vi "S2C_Access_ManageUpdate.vi"(8 "Error In":errorcluster, 10 "Coords":cluster{"Row":i32, "Column":i32}, 11 "ItemTag":string) -> (0 "Error Out":errorcluster)   [LabVIEW 2015]
uses:
  S2C_Access_Globals.vi
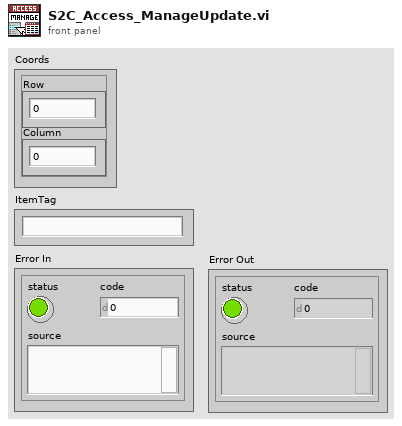
[diagram p1: front panel]
types:
  T1 = cluster{"ItemNames[0]":string, "ItemNames[1]":string, "ItemNames[2]":string}
  T2 = cluster{"[0]":string, "[1]":string, "[2]":string}
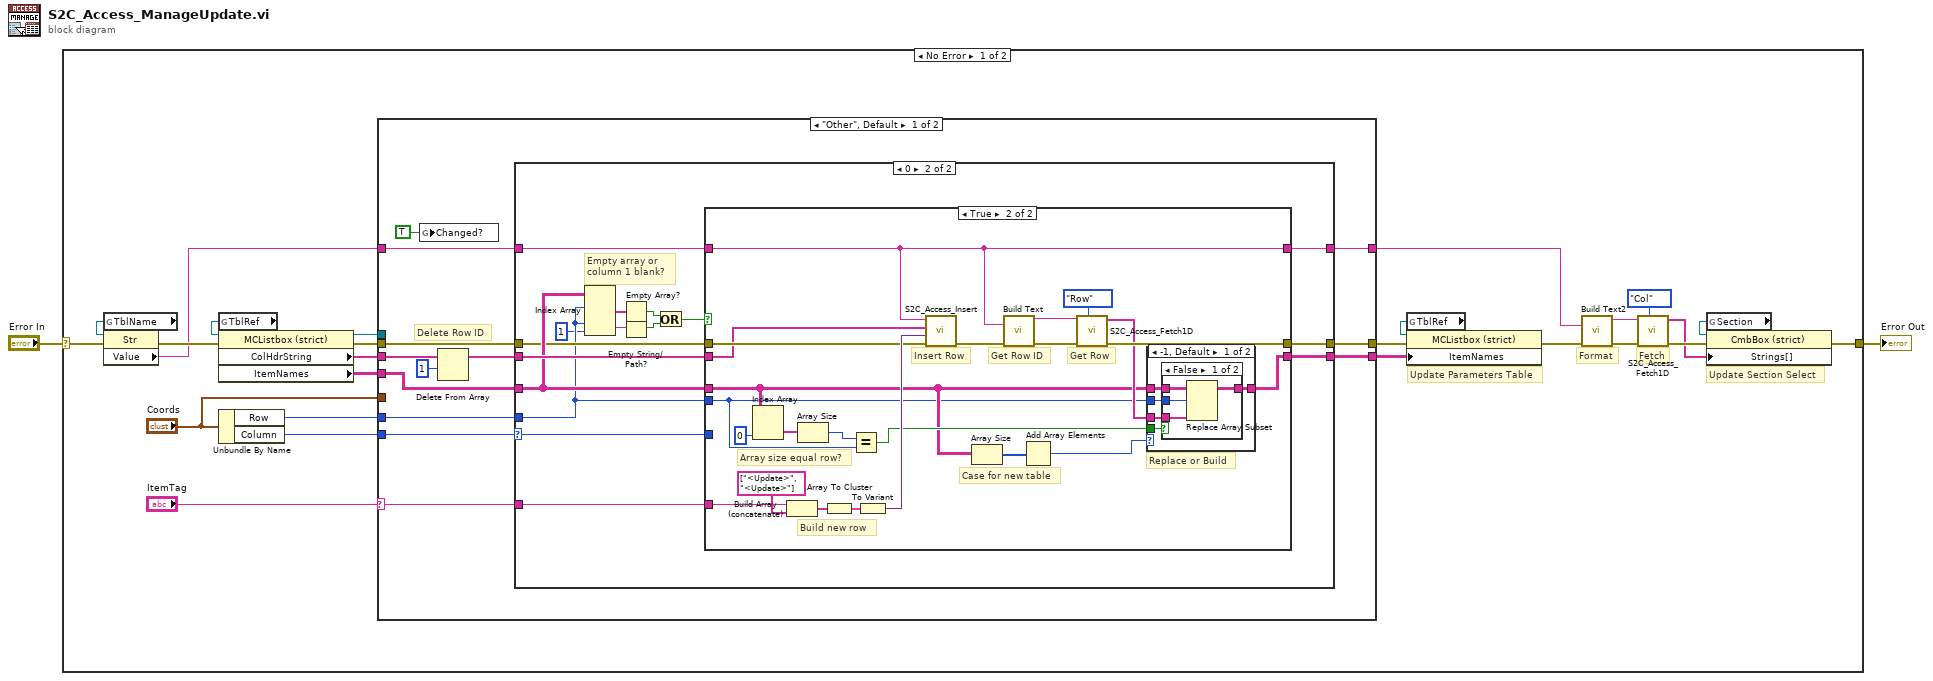
[diagram p0: block diagram]
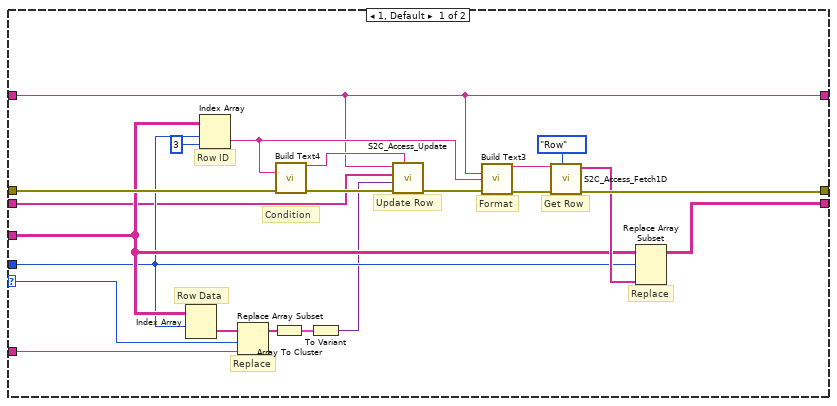
[diagram p2: hidden frame]
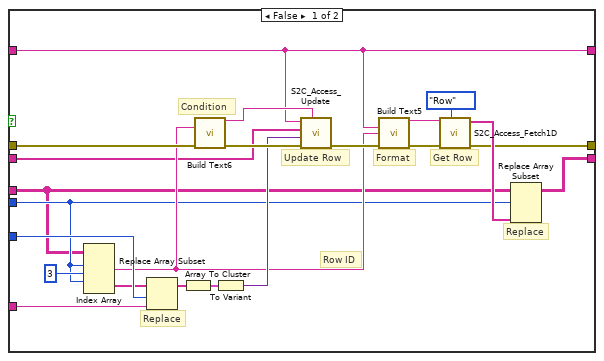
[diagram p3: hidden frame]
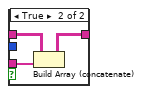
[diagram p4: hidden frame]
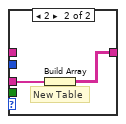
[diagram p5: hidden frame]
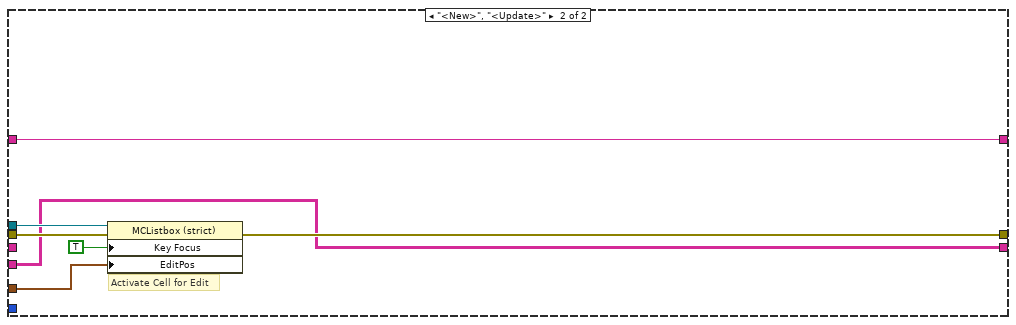
[diagram p6: hidden frame]
diagram:
  n1 = case shown="No Error" "Error In" {
    selector: "Error In" -> [w11 w145]
    tunnel: [w13 w145] -> w1
    frame No Error {
      # "Update Parameters Table"
      # "Update Section Select"
      # "Fetch"
      # "Format"
      n2 = global read "S2C_Access_Globals.vi" "TblName"() -> (w12:refnum<vi>)
      n3 = property class="Str"(reference=w12, error in=w11) -> (error out=w10:errorcluster, "Value"=w9:string)  [unwired: 1 out]
      n4 = global read "S2C_Access_Globals.vi" "TblRef"() -> (w21:refnum<vi>)
      n5 = property class="MCListbox (strict)"(reference=w21, error in=w10) -> (reference out=w22:refnum<vi>, error out=w27:errorcluster, "ColHdrString"=w7:string[], "ItemNames"=w6:string[][])
      n6 = Unbundle By Name("Coords") -> ("Row"=w26:i32, "Column"=w5:i32)
      n7 = case shown="\"Other\", Default" "ItemTag" {
        selector: "ItemTag" -> [w33 _]
        tunnel: w5 -> [w34 _]
        tunnel: w27 -> [w40 w144]
        tunnel: w26 -> [w35 _]
        tunnel: "Coords" -> [_ w142]
        tunnel: w6 -> [w36 w138]
        tunnel: [w39 w138] -> w25
        tunnel: [w38 w140] -> w24
        tunnel: w7 -> [w31 _]
        tunnel: w22 -> [_ w143]
        tunnel: w9 -> [w37 w139]
        tunnel: [w29 w139] -> w3
        frame "Other", Default {
          # "Delete Row ID"
          n8 = global write "S2C_Access_Globals.vi" "Changed?"(TRUE ("Changed?")) -> ()
          n9 = Delete From Array(array=w31, length=1) -> (array with subset deleted=w30:string[])  [unwired: 1 in, 1 out]
          n10 = case shown="0" w34 {
            selector: w34 -> [w47 w71]
            tunnel: w40 -> [w54 w73]
            tunnel: w35 -> [w49 w67]
            tunnel: w36 -> [w50 w75]
            tunnel: [w56 w76] -> w39
            tunnel: [w58 w77] -> w38
            tunnel: w30 -> [w42 w78]
            tunnel: w33 -> [w46 w72]
            tunnel: w37 -> [w41 w74]
            tunnel: [w41 w63] -> w29
            frame 1, Default {
              # "Replace"
              # "Condition"
              # "Row ID"
              # "Format"
              # "Row Data"
              # "Replace"
              # "Get Row"
              # "Update Row"
              n11 = Index Array(array=w50, index (row)=w49) -> (element=w48:string[])  [unwired: 1 in]
              n12 = Index Array(array=w50, index (row)=w49, index (col)=3 ("disabled index (col)")) -> (element=w52:string)
              n13 = Replace Array Subset(array=w48, new element=w46, index=w47) -> (w45:string[])
              n14 = Array To Cluster(array=w45) -> (cluster=w44:T1)
              n15 = call "Build Text4"("ID"=w52, "error in (no error)"=w54) -> ("Result"=w51:string, "error out"=w53:errorcluster)  [unwired: 12 in]
              n16 = To Variant(anything=w44) -> (Variant=w43:variant)
              n17 = call "S2C_Access_Update.vi"("Condition"=w51, "Error In"=w53, "Data"=w43, "Columns"=w42, "Table"=w41) -> ("Error Out"=w55:errorcluster)  [unwired: 6 in]
              n18 = call "Build Text3"("Table"=w41, "ID"=w52, "error in (no error)"=w55) -> ("Result"=w60:string, "error out"=w61:errorcluster)  [unwired: 11 in]
              n19 = call "S2C_Access_Fetch1D.vi"("Selection"=enum16{"Row", "Col"}."Row", "Error In"=w61, "Query"=w60) -> ("Error Out"=w58:errorcluster, "Data"=w57:string[])  [unwired: 7 in]
              n20 = Replace Array Subset(array=w50, new element=w57, index (row)=w49) -> (w56:string[][])  [unwired: 1 in]
            }
            frame 0 {
              # "Empty array or\ncolumn 1 blank?"
              n21 = Index Array(array=w75, index (row) #1=w67, index (row) #2=w67, index (col) #2=1 ("disabled index (col)")) -> (element #1=w66:string[], element #2=w64:string)  [unwired: 1 in]
              n22 = Empty Array?(array=w66) -> (empty?=w70:bool)
              n23 = Empty String/Path?(string/path=w64) -> (empty?=w69:bool)
              n24 = Or(x=w70, y=w69) -> (x .or. y?=w68:bool)
              n25 = case shown="True" w68 {
                tunnel: w78 -> [w80 w108]
                tunnel: [w96 w115] -> w77
                tunnel: [w95 w114] -> w76
                tunnel: w75 -> [w81 w102]
                tunnel: w67 -> [w82 w101]
                tunnel: w74 -> [w79 w109]
                tunnel: w73 -> [w92 w112]
                tunnel: w72 -> [w89 w111]
                tunnel: w71 -> [w90 _]
                tunnel: [w79 w109] -> w63
                frame False {
                  # "Row ID"
                  # "Replace"
                  # "Condition"
                  # "Format"
                  # "Replace"
                  # "Update Row"
                  # "Get Row"
                  n26 = Index Array(array=w81, index (row) #1=w82, index (col) #1=3 ("disabled index (col)"), index (row) #2=w82) -> (element #1=w83:string, element #2=w88:string[])  [unwired: 1 in]
                  n27 = Replace Array Subset(array=w88, new element=w89, index=w90) -> (w87:string[])
                  n28 = Array To Cluster(array=w87) -> (cluster=w86:T1)
                  n29 = call "Build Text6"("ID"=w83, "error in (no error)"=w92) -> ("Result"=w93:string, "error out"=w94:errorcluster)  [unwired: 12 in]
                  n30 = To Variant(anything=w86) -> (Variant=w85:variant)
                  n31 = call "S2C_Access_Update.vi"("Condition"=w93, "Error In"=w94, "Data"=w85, "Columns"=w80, "Table"=w79) -> ("Error Out"=w91:errorcluster)  [unwired: 6 in]
                  n32 = call "Build Text5"("Table"=w79, "ID"=w83, "error in (no error)"=w91) -> ("Result"=w99:string, "error out"=w100:errorcluster)  [unwired: 11 in]
                  n33 = call "S2C_Access_Fetch1D.vi"("Selection"=enum16{"Row", "Col"}."Row", "Error In"=w100, "Query"=w99) -> ("Error Out"=w96:errorcluster, "Data"=w97:string[])  [unwired: 7 in]
                  n34 = Replace Array Subset(array=w81, new element=w97, index (row)=w82) -> (w95:string[][])  [unwired: 1 in]
                }
                frame True {
                  # "Case for new table"
                  # "Build new row"
                  # "Get Row ID"
                  # "Replace or Build"
                  # "Array size equal row?"
                  # "Get Row"
                  # "Insert Row"
                  n35 = Index Array(array=w102, index (col)=0 ("disabled index (col)")) -> (element=w107:string[])  [unwired: 1 in]
                  n36 = Build Array (concatenate)(w111, string[] ["<Update>", "<Update>"]) -> (w122:string[])
                  n37 = Array Size(array=w107) -> (size(s)=w110:i32)
                  n38 = Array To Cluster(array=w122) -> (cluster=w121:T2)
                  n39 = Equal?(x=w110, y=w101) -> (x = y?=w103:bool)
                  n40 = To Variant(anything=w121) -> (Variant=w120:variant)
                  n41 = call "S2C_Access_Insert.vi"("Error In"=w112, "Data"=w120, "Columns"=w108, "Table"=w109) -> ("Error Out"=w119:errorcluster)  [unwired: 7 in]
                  n42 = Array Size(array=w102) -> (size(s)=w105:i32[])
                  n43 = call "Build Text"("Table"=w109, "error in (no error)"=w119) -> ("Result"=w117:string, "error out"=w118:errorcluster)  [unwired: 12 in]
                  n44 = Add Array Elements(numeric array=w105) -> (sum=w104:i32)
                  n45 = call "S2C_Access_Fetch1D.vi"("Selection"=enum16{"Row", "Col"}."Row", "Error In"=w118, "Query"=w117) -> ("Error Out"=w115:errorcluster, "Data"=w113:string[])  [unwired: 7 in]
                  n46 = case shown="-1, Default" w104 {
                    tunnel: [w128 w136] -> w114
                    tunnel: w113 -> [w127 w137]
                    tunnel: w102 -> [w126 _]
                    tunnel: w103 -> [w125 _]
                    tunnel: w101 -> [w124 _]
                    frame -1, Default {
                      n47 = case shown="False" w125 {
                        tunnel: [w132 w135] -> w128
                        tunnel: w127 -> [w131 w133]
                        tunnel: w126 -> [w130 w134]
                        tunnel: w124 -> [w129 _]
                        frame False {
                          n48 = Replace Array Subset(array=w130, new element=w131, index (row)=w129) -> (w132:string[][])  [unwired: 1 in]
                        }
                        frame True {
                          n49 = Build Array (concatenate)(w134, w133) -> (w135:string[][])
                        }
                      }
                    }
                    frame 2 {
                      # "New Table"
                      n50 = Build Array(w137) -> (w136:string[][])
                    }
                  }
                }
              }
            }
          }
        }
        frame "<New>", "<Update>" {
          # "Activate Cell for Edit"
          n51 = property class="MCListbox (strict)"(reference=w143, error in=w144, "Key Focus"=TRUE, "EditPos"=w142) -> (error out=w140:errorcluster)  [unwired: 1 out]
        }
      }
      n52 = global read "S2C_Access_Globals.vi" "TblRef"() -> (w23:refnum<vi>)
      n53 = property class="MCListbox (strict)"(reference=w23, error in=w24, "ItemNames"=w25) -> (error out=w8:errorcluster)  [unwired: 1 out]
      n54 = call "Build Text2"("Table"=w3, "error in (no error)"=w8) -> ("Result"=w18:string, "error out"=w17:errorcluster)  [unwired: 12 in]
      n55 = call "S2C_Access_Fetch1D.vi"("Selection"=enum16{"Row", "Col"}."Col", "Error In"=w17, "Query"=w18) -> ("Error Out"=w15:errorcluster, "Data"=w14:string[])  [unwired: 7 in]
      n56 = global read "S2C_Access_Globals.vi" "Section"() -> (w16:refnum<vi>)
      n57 = property class="CmbBox (strict)"(reference=w16, error in=w15, "Strings[]"=w14) -> (error out=w13:errorcluster)  [unwired: 1 out]
    }
    frame Error {
    }
  }
  "Error Out" <- w1
